vi "Array.vi"() -> ()   [LabVIEW 2020]
panel:
  out "retrn string":string
  out "Cluster":cluster{"Array":dbl[]}
  out "astr2":string
  in  "astr":string
  out "Numeric 2":i32
  in  "Numeric":i32
  out "Array 2":dbl[](array[numeric])
  in  "Array":dbl[](array[numeric])
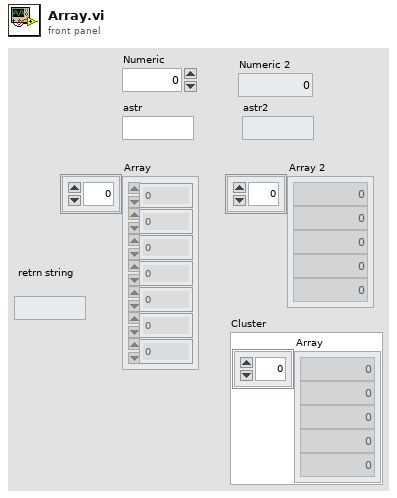
[diagram p1: front panel]
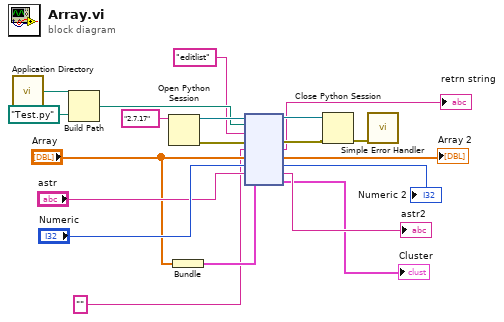
[diagram p0: block diagram]
diagram:
  n1 = call <vilib>:"Application Directory.vi"() -> ("Application Directory"=w15:path)
  n2 = Build Path(base path=w15, name or relative path=path "Test.py") -> (appended path=w13:path)
  n3 = Open Python Session(python version="2.7.17" ("Python version")) -> (session out=w20:refnum<k35>, error out=w19:errorcluster)  [unwired: 2 in]
  n4 = Bundle("Array"="Array") -> (w4:cluster{"Array":dbl[]})  [unwired: 1 in]
  n5 = node(w20, w13, "editlist" ("function name"), w19, "", "Array", "Numeric", "astr", w4) -> (w17:refnum<k35>, w18:errorcluster, →"retrn string":string, →"Array 2":dbl[], →"Numeric 2":i32, →"astr2":string, →"Cluster":cluster{"Array":dbl[]})  [unwired: 2 out]
  n6 = Close Python Session(session in=w17, error in=w18) -> (11:w11:errorcluster)
  n7 = call <vilib>:"Simple Error Handler.vi"("error in (no error)"=w11) -> ()  [unwired: 4 in, 5 out]
